vi "Phasor Calibrate Complex Phasor.vi"(5 "Calibration Phasor":T2, 6 "Force Calibration (T)":bool=TRUE, 7 "Phasor Calibration Map":T3={"Phasor Frequency"=80000000.0, "Calibration Lifetime"=1e-09, "ROI Centers"=[], "ROI Descriptors"=[], "Map Resolution X"=0, "Map Resolution Y"=0, "z Array"=[]} {"ROI Descriptors"."Contours"."Type" items=["No Selection", "Point", "Line", "Rectangle", "Oval", "Polygon", "Freehand Region", "Annulus", "Unused2", "Unused3", "Broken Line", "Freehand Line", "Rotated Rectangle"]}, 8 "Error In":errorcluster, 10 "Calibration Type Used":T1, 11 "Complex Phasor Array (VxH)":csg[][](array[numeric])) -> (0 "Error Out":errorcluster, 3 "Corrected Complex Phasor Array (VxH)":csg[][](array[numeric]), 4 "CPU (s)":dbl)   [LabVIEW 2021, in "Phasor.lvlib"]
uses:
  Phasor.lvlib
  Phasor Calibration Map v2.ctl
  Calibration Phasor (m, phi).ctl
  Phasor Calibration Type.ctl
  32e74294-0381-4c43-9503-00d59542fdb5.vi
  0d129a73-88dd-4982-b217-d040be4adb76.vi
  23ce9f9a-f287-4f49-a714-90e89a71442e.vi
panel:
  # "see the License on the block diagram (Ctrl+E or Window:Show Block Diagram)"
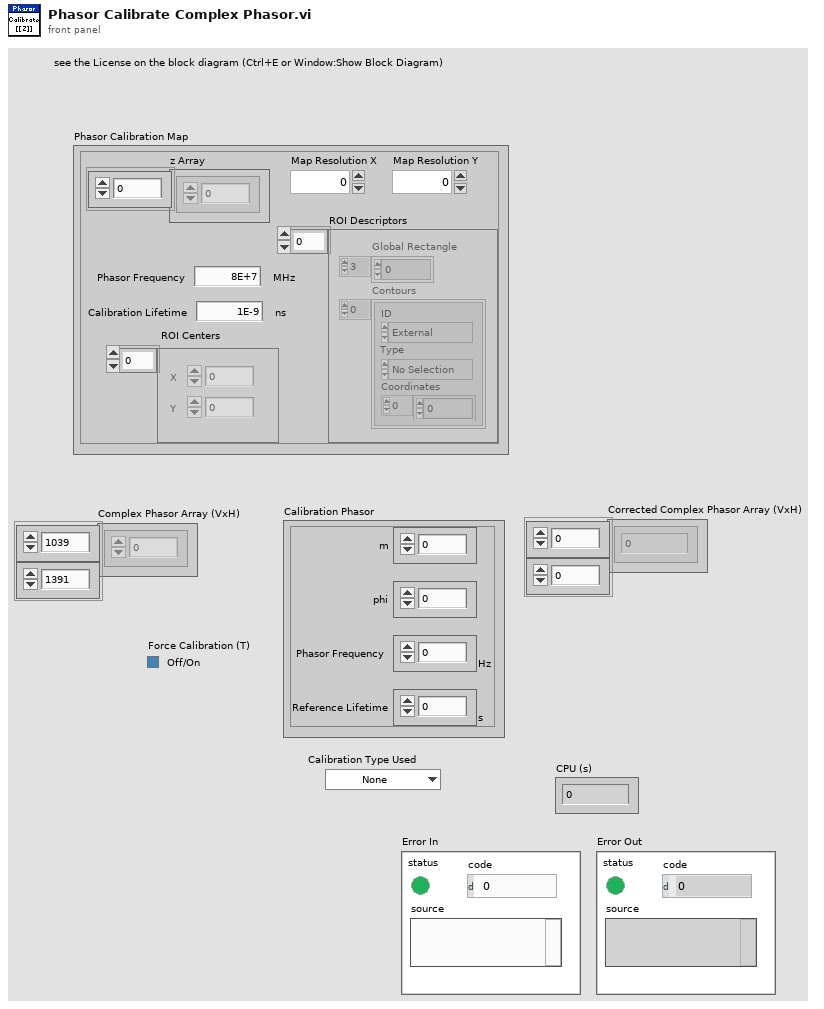
[diagram p1: front panel]
types:
  T1 = typedef "Phasor.lvlib/Phasor Calibration Type.ctl" = enum16{"None", "Single Phasor", "Phasor Series", "Phasor Map"}
  T2 = typedef "Phasor.lvlib/Calibration Phasor (m, phi).ctl" = cluster{"m":dbl, "phi":dbl, "Phasor Frequency":dbl[unit], "Reference Lifetime":dbl[unit]}
  T3 = typedef "Phasor.lvlib/Phasor Calibration Map v2.ctl" = cluster{"Phasor Frequency":dbl[unit], "Calibration Lifetime":dbl[unit], "ROI Centers":cluster{"X":i32, "Y":i32}[], "ROI Descriptors":T4[], "Map Resolution X":i32, "Map Resolution Y":i32, "z Array":cdb[]}
  T4 = typedef "ROI Descriptor" = cluster{"Global Rectangle":i32[], "Contours":cluster{"ID":enum32{"External", "Internal"}, "Type":u32, "Coordinates":i32[]}[]}
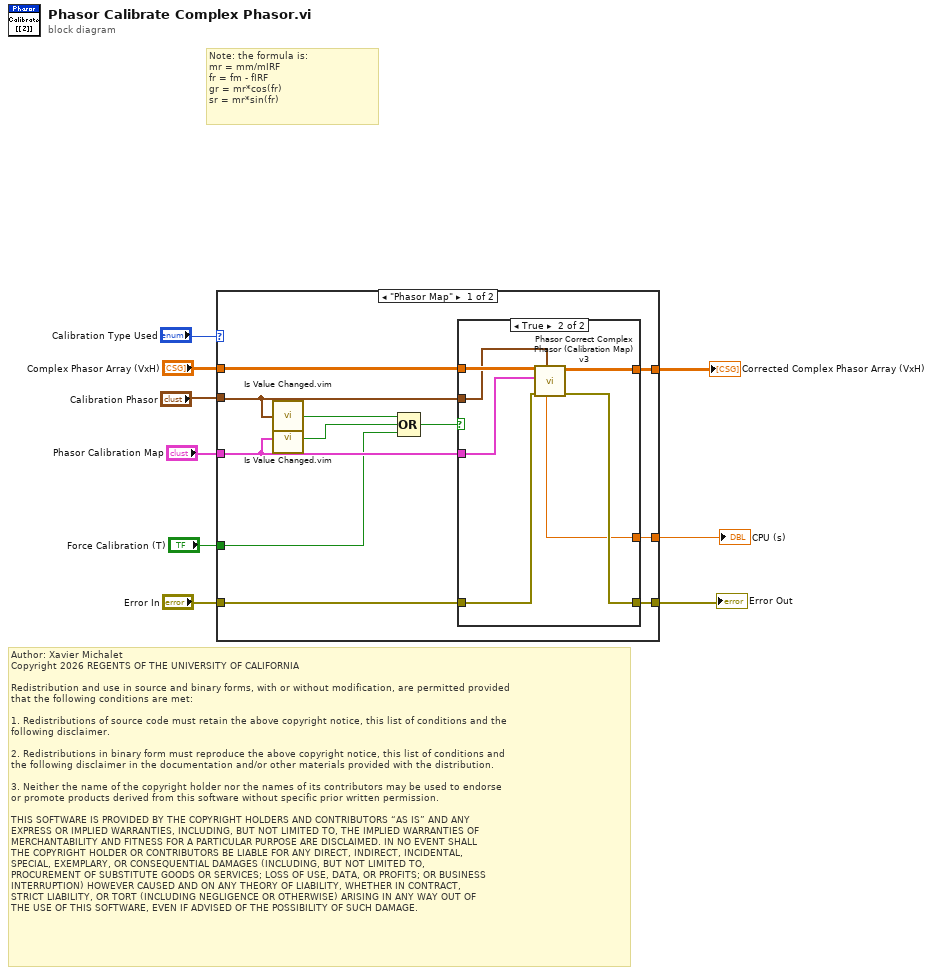
[diagram p0: block diagram]
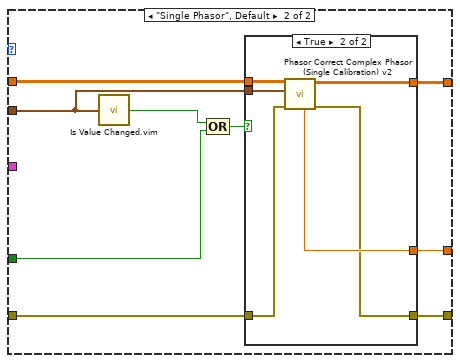
[diagram p3: hidden frame]
diagram:
  # "Author: Xavier Michalet\nCopyright 2026 REGENTS OF THE UNIVERSITY OF CALIFORNIA\n\nRedistribution and use in source and binary forms, with or without modification, are permitted provided\nthat the following conditions are met:\n\n1. Redistributions of source code must retain the above copyright notice, this list of conditions and the\nfollowing disclaimer.\n\n2. Redistributions in binary form must reproduce the above copyright notice, this list of conditions and\nthe following disclaimer in the documentation and/or other materials provided with the distribution.\n\n3. Neither the name of the copyright holder nor the names of its contributors may be used to endorse \nor promote products derived from this software without specific prior written permission.\n\nTHIS SOFTWARE IS PROVIDED BY THE COPYRIGHT HOLDERS AND CONTRIBUTORS “AS IS” AND ANY \nEXPRESS OR IMPLIED WARRANTIES, INCLUDING, BUT NOT LIMITED TO, THE IMPLIED WARRANTIES OF\nMERCHANTABILITY AND FITNESS FOR A PARTICULAR PURPOSE ARE DISCLAIMED. IN NO EVENT SHALL\nTHE COPYRIGHT HOLDER OR CONTRIBUTORS BE LIABLE FOR ANY DIRECT, INDIRECT, INCIDENTAL, \nSPECIAL, EXEMPLARY, OR CONSEQUENTIAL DAMAGES (INCLUDING, BUT NOT LIMITED TO, \nPROCUREMENT OF SUBSTITUTE GOODS OR SERVICES; LOSS OF USE, DATA, OR PROFITS; OR BUSINESS\nINTERRUPTION) HOWEVER CAUSED AND ON ANY THEORY OF LIABILITY, WHETHER IN CONTRACT, \nSTRICT LIABILITY, OR TORT (INCLUDING NEGLIGENCE OR OTHERWISE) ARISING IN ANY WAY OUT OF\nTHE USE OF THIS SOFTWARE, EVEN IF ADVISED OF THE POSSIBILITY OF SUCH DAMAGE."
  # "Note: the formula is:\nmr = mm/mIRF\nfr = fm - fIRF\ngr = mr*cos(fr)\nsr = mr*sin(fr)"
  n1 = case shown="\"Phasor Map\"" "Calibration Type Used" {
    tunnel: "Complex Phasor Array (VxH)" -> [w20 w38]
    tunnel: [w19 w37] -> w7
    tunnel: "Calibration Phasor" -> [w14 w31]
    tunnel: [w16 w36] -> w5
    tunnel: "Phasor Calibration Map" -> [w13 _]
    tunnel: "Error In" -> [w18 w35]
    tunnel: [w17 w34] -> w2
    tunnel: "Force Calibration (T)" -> [w10 w33]
    frame "Phasor Map" {
      n2 = call "Is Value Changed.vim"("value"=w14) -> ("changed or first call?"=w12:bool)
      n3 = call "Is Value Changed.vim"("value"=w13) -> ("changed or first call?"=w11:bool)
      n4 = Compound Arithmetic op=OR(w12, w11, w10) -> (w15:bool)
      n5 = case shown="True" w15 {
        tunnel: w20 -> [w22 w29]
        tunnel: [w22 w28] -> w19
        tunnel: w18 -> [w21 w27]
        tunnel: [w21 w26] -> w17
        tunnel: [_ w25] -> w16
        tunnel: w14 -> [_ w24]
        tunnel: w13 -> [_ w23]
        frame False {
        }
        frame True {
          n6 = call "Phasor Correct Complex Phasor (Calibration Map) v3.vi"("Calibration Phasor"=w24, "Error In"=w27, "Phasor Calibration Map"=w23, "Complex Phasor Array (VxH)"=w29) -> ("Error Out"=w26:errorcluster, "Corrected Complex Phasor Array (VxH)"=w28:csg[][], "CPU (s)"=w25:dbl)  [unwired: 5 in]
        }
      }
    }
    frame "Single Phasor", Default {
      n7 = call "Is Value Changed.vim"("value"=w31) -> ("changed or first call?"=w30:bool)
      n8 = Compound Arithmetic op=OR(w30, w33) -> (w32:bool)
      n9 = case shown="True" w32 {
        tunnel: w38 -> [w40 w46]
        tunnel: [w40 w45] -> w37
        tunnel: [_ w44] -> w36
        tunnel: w35 -> [w39 w43]
        tunnel: [w39 w42] -> w34
        tunnel: w31 -> [_ w41]
        frame False {
        }
        frame True {
          n10 = call "Phasor Correct Complex Phasor (Single Calibration) v2.vi"("Error In"=w43, "Calibration Phasor (m, phi, f, t0)"=w41, "Complex Phasor Array (V x H)"=w46) -> ("Error Out"=w42:errorcluster, "Corrected Complex Phasor Array (V x H)"=w45:csg[][], "CPU (s)"=w44:dbl)  [unwired: 6 in]
        }
      }
    }
  }
  "Corrected Complex Phasor Array (VxH)" <- w7
  "Error Out" <- w2
  "CPU (s)" <- w5
